vi "ManageGradientSearchRoutines.vi"(0 "System no.":i32=1 min=1 step=1, 5 "error in (no error)":errorcluster) -> (19 "error out":errorcluster)   [LabVIEW 2020]
doc: "This VI allows to add or edit Gradient Search Routines (FDG).\n\nRoutines can be managed on the controller directly or via text files."
uses:
  Message Cluster.ctl
  <vilib>/Utility/miscctls.llb/LVRowAndColumnTypeDef.ctl
panel:
  in  "Update from selected":bool
  in  "Name":string
  in  "Send to controller":bool
  in  "Board":i32 min=1 max=5 step=1
  in  "Minimum Level":dbl format="%.3f"
  in  "Speed offset":dbl format="%.4f"
  in  "Max. dir. changes":i32
  in  "Speed factor":dbl format="%.4f"
  in  "Max velocity":dbl format="%.4f"
  in  "Frequency":dbl format="%.3f"
  in  "Max amplitude":dbl format="%.4f"
  in  "Min amplitude":dbl format="%.4f"
  in  "Step axis":string
  in  "Scan axis":string
  in  "stop":bool
  in  "Available Routines":string[][](table)
  # "Routine definition"
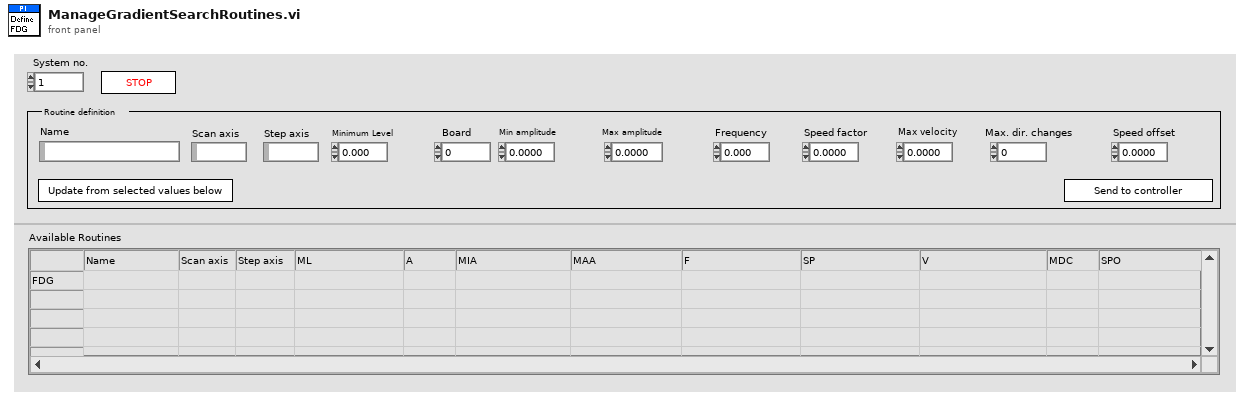
[diagram p1: front panel]
types:
  T1 = typedef "Message Cluster.ctl" = cluster{"Message":string, "Message Data":variant}
  T2 = cluster{"Set speed factor?":bool, "Speed factor":dbl}
  T3 = cluster{"Set max. velocity?":bool, "Max velocity":dbl}
  T4 = cluster{"Set max. dir. changes?":bool, "Max. dir. changes":i32}
  T5 = cluster{"Set speed offset?":bool, "Speed offset":dbl}
  T6 = cluster{"Min amplitude":dbl, "Set min. amplitude?":bool, "Max amplitude":dbl, "Set max. amplitude?":bool}
  T7 = typedef "LVRowAndColumnTypeDef.ctl" = cluster{"Row":i32, "Column":i32}
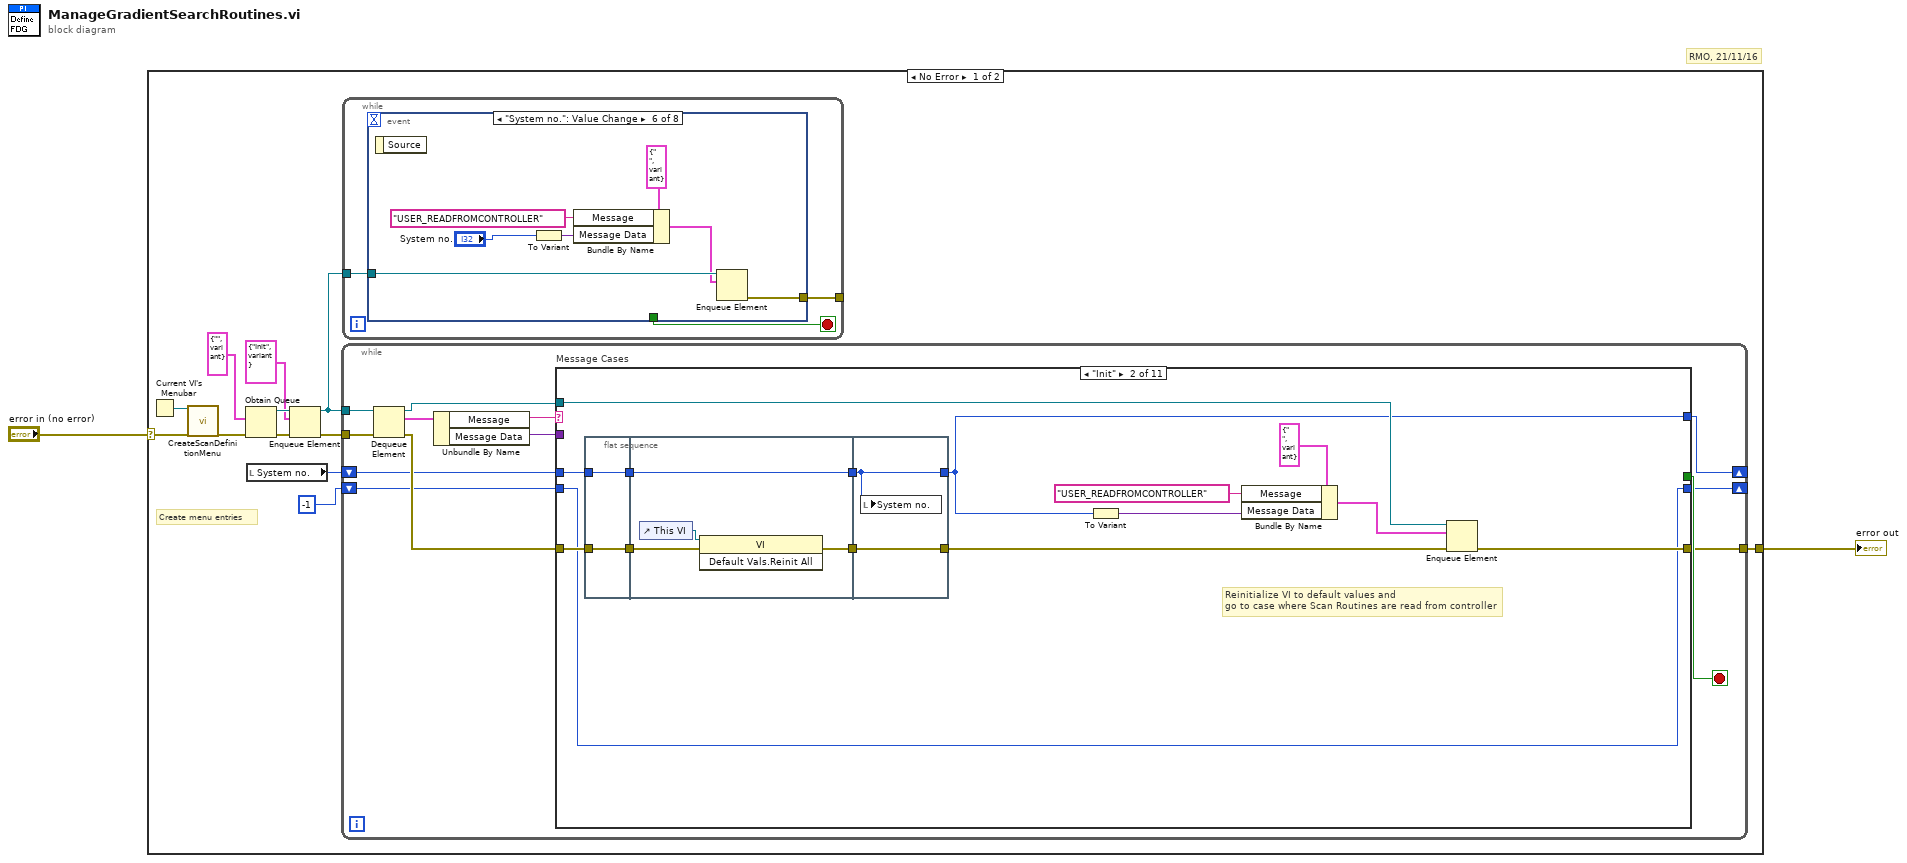
[diagram p0: block diagram]
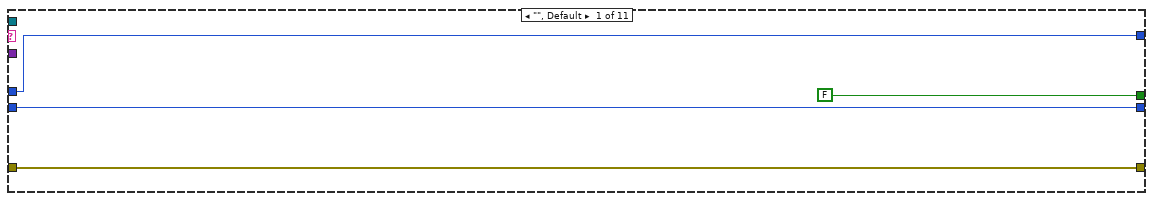
[diagram p2: hidden frame]
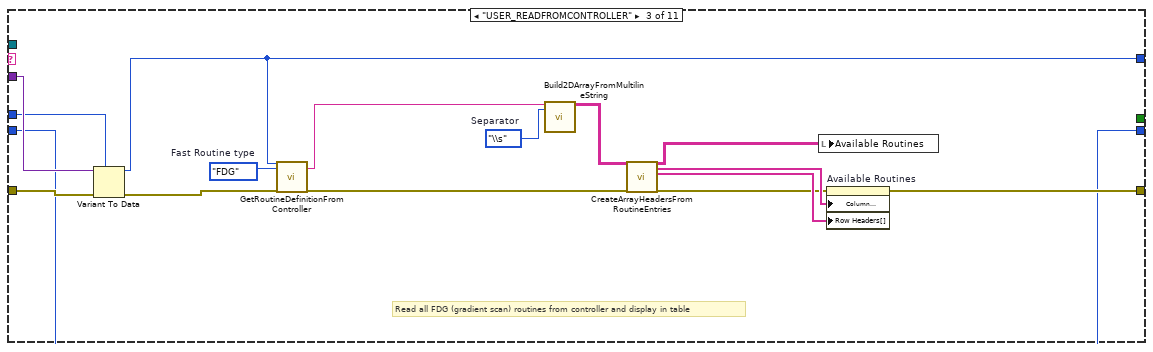
[diagram p3: hidden frame]
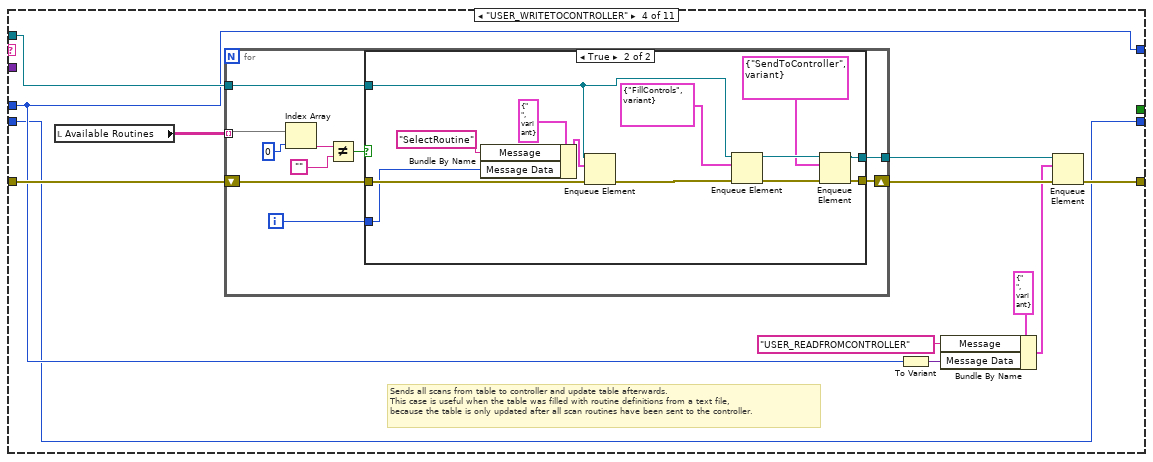
[diagram p4: hidden frame]
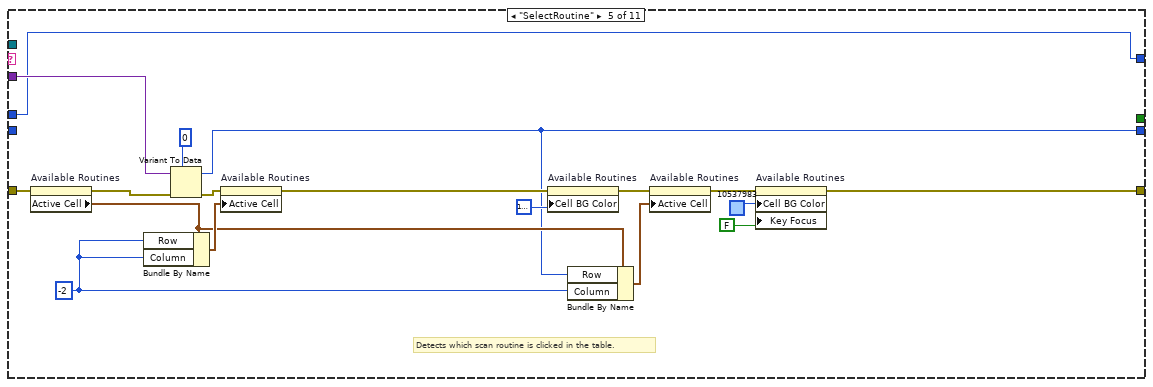
[diagram p6: hidden frame]
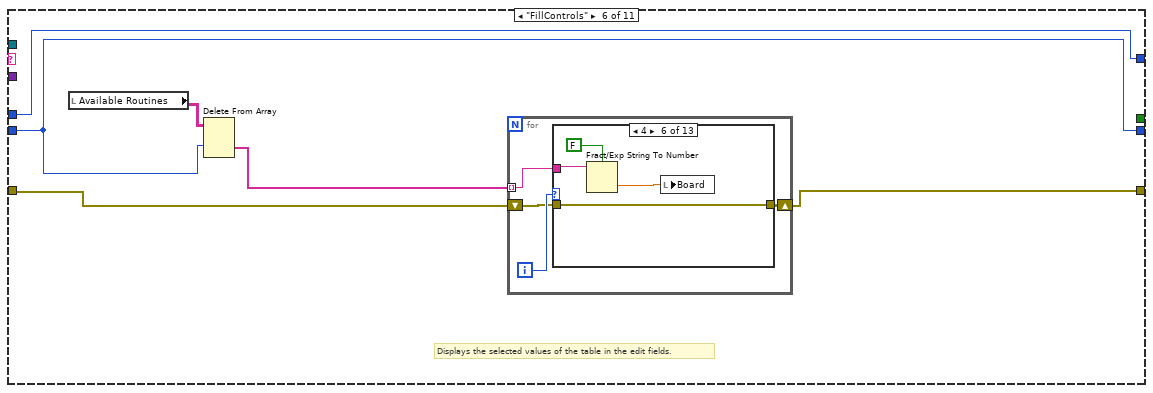
[diagram p7: hidden frame]
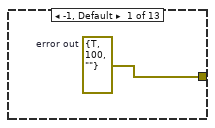
[diagram p8: hidden frame]
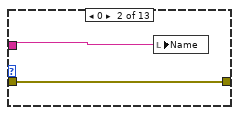
[diagram p9: hidden frame]
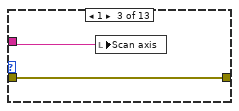
[diagram p10: hidden frame]
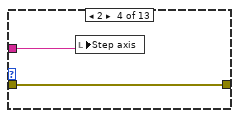
[diagram p11: hidden frame]
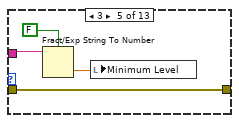
[diagram p12: hidden frame]
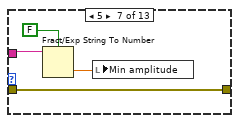
[diagram p13: hidden frame]
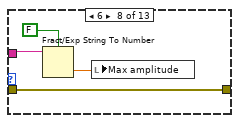
[diagram p14: hidden frame]
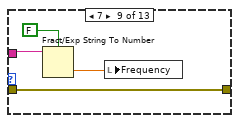
[diagram p15: hidden frame]
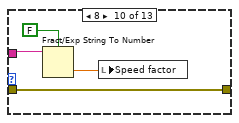
[diagram p16: hidden frame]
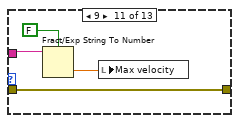
[diagram p17: hidden frame]
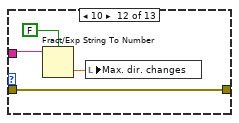
[diagram p18: hidden frame]
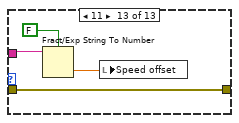
[diagram p19: hidden frame]
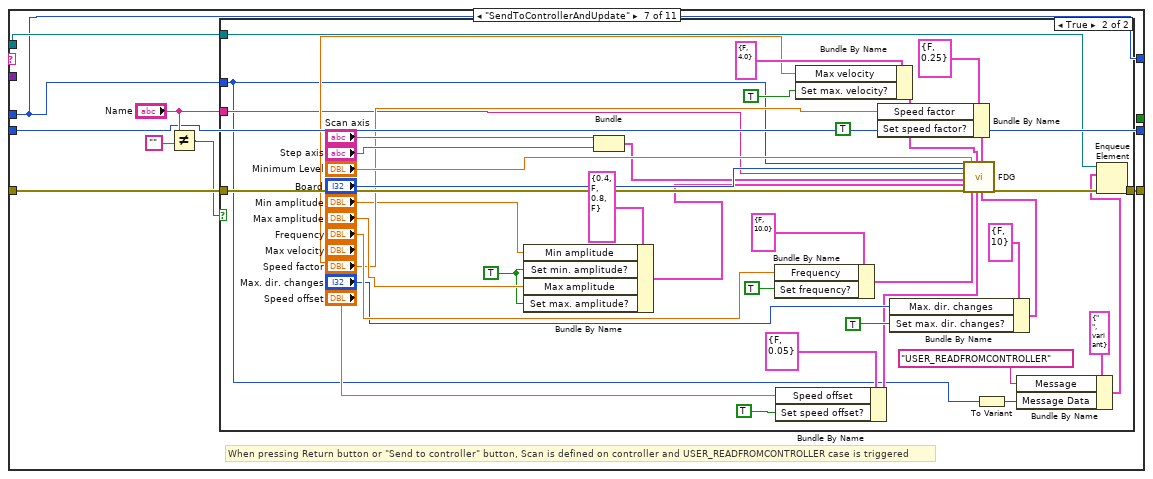
[diagram p20: hidden frame]
diagram:
  # "RMO, 21/11/16"
  n1 = case shown="No Error" "error in (no error)" {
    selector: "error in (no error)" -> [w5 w330]
    tunnel: [w6 w330] -> w2
    frame No Error {
      # "Create menu entries"
      n2 = Current VI's Menubar() -> (w7:refnum<k9>)
      n3 = call "CreateScanDefinitionMenu.vi"("menu reference"=w7, "error in (no error)"=w5) -> ("error out"=w8:errorcluster)  [unwired: 17 out]
      n4 = Obtain Queue(element data type=T1 {"Message"="", "Message Data"=variant} ("Message Cluster"), error in (no error)=w8) -> (queue out=w12:refnum<queue>, error out=w13:errorcluster)  [unwired: 2 in, 2 out]
      n5 = local read "System no."() -> (w4:i32)
      n6 = Enqueue Element(queue=w12, element=T1 {"Message"="Init", "Message Data"=variant}, error in (no error)=w13) -> (queue out=w9:refnum<queue>, error out=w10:errorcluster)  [unwired: 2 out]
      n7 = while {
        tunnel: w10 -> [w27]
        tunnel: w9 -> [w26]
        tunnel: [w21] -> w6
        shift-right: [w17] -> _
        shift-left: w4 -> [w20]
        shift-right: [w16] -> _
        shift-left: -1 ("Horizontal") -> [w15]
        stop <- w22 stop-if-true
        n8 = Dequeue Element(queue=w26, error in (no error)=w27) -> (queue out=w18:refnum<queue>, element=w25:T1, error out=w24:errorcluster)  [unwired: 2 out]
        n9 = Unbundle By Name(w25) -> ("Message"=w23:string, "Message Data"=w19:variant)
        n10 = case "Message Cases" shown="\"Init\"" w23 {
          tunnel: w24 -> [w31 w44 w61 w80 w123 w126 w186 w262 w268 w274 w286]
          tunnel: [w31 w45 w64 w78 w109 w129 w185 w242 w265 w276 w287] -> w21
          tunnel: [FALSE _ _ _ _ _ _ _ _ _ TRUE] -> w22
          tunnel: w20 -> [w29 w37 w58 w72 w110 w128 w180 w229 w264 w272 w283]
          tunnel: w19 -> [_ _ w59 _ w125 _ _ _ _ _ _]
          tunnel: w18 -> [_ w46 _ w81 _ _ w184 _ _ _ _]
          tunnel: [w29 w32 w57 w72 w110 w128 w180 w229 w264 w272 w283] -> w17
          tunnel: [w28 w38 w56 w71 w108 w127 w179 w228 w263 w271 w282] -> w16
          tunnel: w15 -> [w28 w38 w56 w71 _ w127 w179 w228 w263 w271 w282]
          frame "", Default {
          }
          frame "Init" {
            # "Reinitialize VI to default values and\ngo to case where Scan Routines are read from controller"
            n11 = flat-sequence {
              tunnel: w37 -> [w47]
              tunnel: w44 -> [w48]
              tunnel: [w48] -> w36
              tunnel: [w47] -> w35
              tunnel: w36 -> [w51]
              tunnel: w35 -> [w49]
              tunnel: [w50] -> w34
              tunnel: [w49] -> w33
              tunnel: [w54] -> w43
              tunnel: w34 -> [w54]
              tunnel: w33 -> [w53]
              tunnel: [w53] -> w32
              frame #0 {
              }
              frame #1 {
                n12 = control-ref of="This VI"() -> (w52:refnum<vi>)
                n13 = invoke class="VI" method="Default Vals.Reinit All"(reference=w52, error in=w51) -> (error out=w50:errorcluster)  [unwired: 1 in, 2 out]
              }
              frame #2 {
                n14 = local write "System no."(w53) -> ()
              }
            }
            n15 = To Variant(anything=w32) -> (Variant=w42:variant)
            n16 = Bundle By Name(cluster=T1 {"Message"="  ", "Message Data"=variant} ("Message Cluster"), "Message"="USER_READFROMCONTROLLER", "Message Data"=w42) -> (w39:T1)
            n17 = Enqueue Element(queue=w46, element=w39, error in (no error)=w43) -> (error out=w45:errorcluster)  [unwired: 3 out]
          }
          frame "USER_READFROMCONTROLLER" {
            w69 = enum16{"\\s", "\\t"}."\\s"  # Separator
            w70 = enum16{"FDG", "FDR"}."FDG"  # Fast Routine type
            # "Read all FDG (gradient scan) routines from controller and display in table"
            n18 = Variant To Data(error in=w61, type=w58, Variant=w59) -> (data=w57:i32, error out=w60:errorcluster)
            n19 = call "GetRoutineDefinitionFromController.vi"("System no."=w57, "Fast Routine type"=w70, "error in"=w60) -> ("Routine Definitons"=w55:string, "error out"=w63:errorcluster)  [unwired: 15 out]
            n20 = call "Build2DArrayFromMultilineString.vi"("String"=w55, "Separator"=w69) -> ("2D Array out"=w68:string[][])  [unwired: 17 out]
            n21 = call "CreateArrayHeadersFromRoutineEntries.vi"("Available Routines"=w68, "error in"=w63) -> ("Available Routines out"=w67:string[][], "Column Headers"=w66:string[], "Row Headers"=w65:string[], "error out"=w62:errorcluster)  [unwired: 14 out]
            n22 = local write "Available Routines"(w67) -> ()
            n23 = property on="Available Routines" class="Tbl (strict)"(error in=w62, "Column Headers[]"=w66, "Row Headers[]"=w65) -> (error out=w64:errorcluster)  [unwired: 1 in, 1 out]
          }
          frame "USER_WRITETOCONTROLLER" {
            # "Sends all scans from table to controller and update table afterwards.\nThis case is useful when the table was filled with routine definitions from a text file,\nbecause the table is only updated after all scan routines have been sent to the controller."
            n24 = local read "Available Routines"() -> (w82:string[][])
            n25 = for {
              tunnel: w82 -> [w88] mode=indexing
              tunnel: w81 -> [w91]
              shift-right: [w89] -> w79
              shift-left: w80 -> [w90]
              tunnel: [w83] -> w77
              i -> [w92]
              n26 = Index Array(array=w88, index=0) -> (element=w86:string)
              n27 = Not Equal?(x=w86, y="") -> (x != y?=w84:bool)
              n28 = case shown="True" w84 {
                tunnel: w92 -> [_ w96]
                tunnel: w91 -> [w93 w99]
                tunnel: w90 -> [w94 w101]
                tunnel: [w94 w103] -> w89
                tunnel: [w93 w102] -> w83
                frame False {
                }
                frame True {
                  n29 = Bundle By Name(cluster=T1 {"Message"="  ", "Message Data"=variant} ("Message Cluster"), "Message"="SelectRoutine", "Message Data"=w96) -> (w95:T1)
                  n30 = Enqueue Element(queue=w99, element=w95, error in (no error)=w101) -> (error out=w100:errorcluster)  [unwired: 3 out]
                  n31 = Enqueue Element(queue=w99, element=T1 {"Message"="FillControls", "Message Data"=variant} ("Message Cluster"), error in (no error)=w100) -> (queue out=w105:refnum<queue>, error out=w106:errorcluster)  [unwired: 2 out]
                  n32 = Enqueue Element(queue=w105, element=T1 {"Message"="SendToController", "Message Data"=variant}, error in (no error)=w106) -> (queue out=w102:refnum<queue>, error out=w103:errorcluster)  [unwired: 2 out]
                }
              }
            }
            n33 = To Variant(anything=w72) -> (Variant=w76:variant)
            n34 = Bundle By Name(cluster=T1 {"Message"="  ", "Message Data"=variant} ("Message Cluster"), "Message"="USER_READFROMCONTROLLER", "Message Data"=w76) -> (w74:T1)
            n35 = Enqueue Element(queue=w77, element=w74, error in (no error)=w79) -> (error out=w78:errorcluster)  [unwired: 3 out]
          }
          frame "SelectRoutine" {
            w115 = -2 ("Row")
            # "Detects which scan routine is clicked in the table."
            n36 = property on="Available Routines" class="Tbl (strict)"(error in=w123) -> (error out=w111:errorcluster, "Active Cell"=w116:T7)  [unwired: 1 in, 1 out]
            n37 = Bundle By Name(cluster=w116, "Row"=w115, "Column"=w115) -> (w120:T7)
            n38 = Variant To Data(error in=w111, type=0 ("Horizontal"), Variant=w125) -> (data=w108:i32, error out=w122:errorcluster)
            n39 = property on="Available Routines" class="Tbl (strict)"(error in=w122, "Active Cell"=w120) -> (error out=w121:errorcluster)  [unwired: 1 in, 1 out]
            n40 = property on="Available Routines" class="Tbl (strict)"(error in=w121, "Cell BG Color"=u32 16777225 ("Color Box")) -> (error out=w119:errorcluster)  [unwired: 1 in, 1 out]
            n41 = Bundle By Name(cluster=w116, "Row"=w108, "Column"=w115) -> (w114:T7)
            n42 = property on="Available Routines" class="Tbl (strict)"(error in=w119, "Active Cell"=w114) -> (error out=w118:errorcluster)  [unwired: 1 in, 1 out]
            n43 = property on="Available Routines" class="Tbl (strict)"(error in=w118, "Cell BG Color"=u32 10537983 ("Color Box"), "Key Focus"=FALSE) -> (error out=w109:errorcluster)  [unwired: 1 in, 1 out]
          }
          frame "FillControls" {
            # "Displays the selected values of the table in the edit fields."
            n44 = local read "Available Routines"() -> (w131:string[][])
            n45 = Delete From Array(array=w131, index (row)=w127) -> (deleted portion=w130:string[])  [unwired: 2 in, 1 out]
            n46 = for {
              tunnel: w130 -> [w135] mode=indexing
              shift-right: [w132] -> w129
              shift-left: w126 -> [w133]
              i -> [w134]
              n47 = case shown="4" w134 {
                tunnel: w135 -> [_ w137 w140 w142 w145 w149 w153 w157 w161 w165 w169 w173 w177]
                tunnel: w133 -> [_ w138 w139 w141 w146 w150 w154 w158 w162 w166 w170 w174 w178]
                tunnel: [w136 w138 w139 w141 w146 w150 w154 w158 w162 w166 w170 w174 w178] -> w132
                frame -1, Default {
                  w136 = errorcluster {"status"=TRUE, "code"=100, "source"=""}  # error out
                }
                frame 0 {
                  n48 = local write "Name"(w137) -> ()
                }
                frame 1 {
                  n49 = local write "Scan axis"(w140) -> ()
                }
                frame 2 {
                  n50 = local write "Step axis"(w142) -> ()
                }
                frame 3 {
                  n51 = Fract/Exp String To Number(use system decimal point (T)=FALSE, string=w145) -> (number=w144:dbl)  [unwired: 3 out]
                  n52 = local write "Minimum Level"(w144) -> ()
                }
                frame 4 {
                  n53 = Fract/Exp String To Number(use system decimal point (T)=FALSE, string=w149) -> (number=w148:dbl)  [unwired: 3 out]
                  n54 = local write "Board"(w148) -> ()
                }
                frame 5 {
                  n55 = Fract/Exp String To Number(use system decimal point (T)=FALSE, string=w153) -> (number=w152:dbl)  [unwired: 3 out]
                  n56 = local write "Min amplitude"(w152) -> ()
                }
                frame 6 {
                  n57 = Fract/Exp String To Number(use system decimal point (T)=FALSE, string=w157) -> (number=w156:dbl)  [unwired: 3 out]
                  n58 = local write "Max amplitude"(w156) -> ()
                }
                frame 7 {
                  n59 = Fract/Exp String To Number(use system decimal point (T)=FALSE, string=w161) -> (number=w160:dbl)  [unwired: 3 out]
                  n60 = local write "Frequency"(w160) -> ()
                }
                frame 8 {
                  n61 = Fract/Exp String To Number(use system decimal point (T)=FALSE, string=w165) -> (number=w164:dbl)  [unwired: 3 out]
                  n62 = local write "Speed factor"(w164) -> ()
                }
                frame 9 {
                  n63 = Fract/Exp String To Number(use system decimal point (T)=FALSE, string=w169) -> (number=w168:dbl)  [unwired: 3 out]
                  n64 = local write "Max velocity"(w168) -> ()
                }
                frame 10 {
                  n65 = Fract/Exp String To Number(use system decimal point (T)=FALSE, string=w173) -> (number=w172:dbl)  [unwired: 3 out]
                  n66 = local write "Max. dir. changes"(w172) -> ()
                }
                frame 11 {
                  n67 = Fract/Exp String To Number(use system decimal point (T)=FALSE, string=w177) -> (number=w176:dbl)  [unwired: 3 out]
                  n68 = local write "Speed offset"(w176) -> ()
                }
              }
            }
          }
          frame "SendToControllerAndUpdate" {
            # "When pressing Return button or \"Send to controller\" button, Scan is defined on controller and USER_READFROMCONTROLLER case is triggered"
            n69 = Not Equal?(x="Name", y="") -> (x != y?=w182:bool)
            n70 = case shown="True" w182 {
              tunnel: w186 -> [w187 w227]
              tunnel: w180 -> [_ w188]
              tunnel: [w187 w196] -> w185
              tunnel: w184 -> [_ w195]
              tunnel: "Name" -> [_ w193]
              frame False {
              }
              frame True {
                w218 = TRUE
                n71 = Bundle By Name(cluster=T6 {"Min amplitude"=0.4, "Set min. amplitude?"=FALSE, "Max amplitude"=0.8, "Set max. amplitude?"=FALSE} ("Amplitude settings"), "Min amplitude"="Min amplitude", "Set min. amplitude?"=w218, "Max amplitude"="Max amplitude", "Set max. amplitude?"=w218) -> (w220:T6)
                n72 = Bundle("Scan axis"="Scan axis", "Step axis"="Step axis") -> (w222:cluster{"Scan axis":string, "Step axis":string})  [unwired: 1 out]
                n73 = Bundle By Name(cluster=cluster{"Set frequency?":bool, "Frequency":dbl} {"Set frequency?"=FALSE, "Frequency"=10.0} ("Frequency settings"), "Frequency"="Frequency", "Set frequency?"=TRUE) -> (w216:cluster{"Set frequency?":bool, "Frequency":dbl})
                n74 = Bundle By Name(cluster=T5 {"Set speed offset?"=FALSE, "Speed offset"=0.05} ("Speed offset settings"), "Speed offset"="Speed offset", "Set speed offset?"=TRUE) -> (w207:T5)
                n75 = Bundle By Name(cluster=T3 {"Set max. velocity?"=FALSE, "Max velocity"=4.0} ("Velocity settings"), "Max velocity"="Max velocity", "Set max. velocity?"=TRUE) -> (w203:T3)
                n76 = Bundle By Name(cluster=T2 {"Set speed factor?"=FALSE, "Speed factor"=0.25} ("Speed factor settings"), "Speed factor"="Speed factor", "Set speed factor?"=TRUE) -> (w204:T2)
                n77 = Bundle By Name(cluster=T4 {"Set max. dir. changes?"=FALSE, "Max. dir. changes"=10} ("Max. direction changes settings"), "Max. dir. changes"="Max. dir. changes", "Set max. dir. changes?"=TRUE) -> (w213:T4)
                n78 = call "FDG.vi"("System no."=w188, "Board"="Board", "Routinename"=w193, "Axis settings"=w222, "Amplitude settings"=w220, "error in"=w227, "Minimum Level"="Minimum Level", "Frequency settings"=w216, "Velocity settings"=w203, "Speed offset settings"=w207, "Speed factor settings"=w204, "Max. direction changes settings"=w213) -> ("error out"=w197:errorcluster)  [unwired: 7 out]
                n79 = To Variant(anything=w188) -> (Variant=w190:variant)
                n80 = Bundle By Name(cluster=T1 {"Message"="  ", "Message Data"=variant} ("Message Cluster"), "Message"="USER_READFROMCONTROLLER", "Message Data"=w190) -> (w189:T1)
                n81 = Enqueue Element(queue=w195, element=w189, error in (no error)=w197) -> (error out=w196:errorcluster)  [unwired: 3 out]
              }
            }
          }
          frame "SendToController" {
            w258 = TRUE
            # "Defines gradient scan routine on controller."
            n82 = local read "Max. dir. changes"() -> (w232:i32)
            n83 = local read "Minimum Level"() -> (w239:dbl)
            n84 = local read "Max amplitude"() -> (w236:dbl)
            n85 = local read "Min amplitude"() -> (w237:dbl)
            n86 = local read "Max velocity"() -> (w234:dbl)
            n87 = local read "Speed factor"() -> (w233:dbl)
            n88 = local read "Speed offset"() -> (w231:dbl)
            n89 = local read "Frequency"() -> (w235:dbl)
            n90 = local read "Scan axis"() -> (w241:string)
            n91 = local read "Step axis"() -> (w240:string)
            n92 = local read "Name"() -> (w230:string)
            n93 = local read "Board"() -> (w238:i32)
            n94 = Bundle By Name(cluster=T6 {"Min amplitude"=0.4, "Set min. amplitude?"=FALSE, "Max amplitude"=0.8, "Set max. amplitude?"=FALSE} ("Amplitude settings"), "Min amplitude"=w237, "Set min. amplitude?"=w258, "Max amplitude"=w236, "Set max. amplitude?"=w258) -> (w259:T6)
            n95 = Bundle("Scan axis"=w241, "Step axis"=w240) -> (w261:cluster{"Scan axis":string, "Step axis":string})  [unwired: 1 out]
            n96 = Bundle By Name(cluster=cluster{"Set frequency?":bool, "Frequency":dbl} {"Set frequency?"=FALSE, "Frequency"=10.0} ("Frequency settings"), "Frequency"=w235, "Set frequency?"=TRUE) -> (w256:cluster{"Set frequency?":bool, "Frequency":dbl})
            n97 = Bundle By Name(cluster=T5 {"Set speed offset?"=FALSE, "Speed offset"=0.05} ("Speed offset settings"), "Speed offset"=w231, "Set speed offset?"=TRUE) -> (w250:T5)
            n98 = Bundle By Name(cluster=T3 {"Set max. velocity?"=FALSE, "Max velocity"=4.0} ("Velocity settings"), "Max velocity"=w234, "Set max. velocity?"=TRUE) -> (w246:T3)
            n99 = Bundle By Name(cluster=T2 {"Set speed factor?"=FALSE, "Speed factor"=0.25} ("Speed factor settings"), "Speed factor"=w233, "Set speed factor?"=TRUE) -> (w247:T2)
            n100 = Bundle By Name(cluster=T4 {"Set max. dir. changes?"=FALSE, "Max. dir. changes"=10} ("Max. direction changes settings"), "Max. dir. changes"=w232, "Set max. dir. changes?"=TRUE) -> (w254:T4)
            n101 = call "FDG.vi"("System no."=w229, "Board"=w238, "Routinename"=w230, "Axis settings"=w261, "Amplitude settings"=w259, "error in"=w262, "Minimum Level"=w239, "Frequency settings"=w256, "Velocity settings"=w246, "Speed offset settings"=w250, "Speed factor settings"=w247, "Max. direction changes settings"=w254) -> ("error out"=w242:errorcluster)  [unwired: 7 out]
          }
          frame "USER_SAVETOFILE" {
            w269 = enum16{"FDG", "FDR"}."FDG"  # Fast Routine type
            # "Saves all FDG routines to text file."
            n102 = call "GetRoutineDefinitionFromController.vi"("System no."=w264, "Fast Routine type"=w269, "error in"=w268) -> ("Routine Definitons"=w266:string, "error out"=w267:errorcluster)  [unwired: 15 out]
            n103 = Write to Text File(text=w266, error in=w267) -> (error out=w265:errorcluster)  [unwired: 4 out]
          }
          frame "USER_LOADFROMFILE" {
            w281 = enum16{"\\s", "\\t"}."\\s"  # Separator
            # "Load all gradient scan routines from text file and display in table"
            n104 = Read from Text File(error in=w274) -> (text=w270:string, error out=w273:errorcluster)  [unwired: 5 out]
            n105 = call "Build2DArrayFromMultilineString.vi"("String"=w270, "Separator"=w281) -> ("2D Array out"=w280:string[][])  [unwired: 17 out]
            n106 = call "CreateArrayHeadersFromRoutineEntries.vi"("Available Routines"=w280, "error in"=w273) -> ("Available Routines out"=w279:string[][], "Column Headers"=w278:string[], "Row Headers"=w277:string[], "error out"=w275:errorcluster)  [unwired: 14 out]
            n107 = local write "Available Routines"(w279) -> ()
            n108 = property on="Available Routines" class="Tbl (strict)"(error in=w275, "Column Headers[]"=w278, "Row Headers[]"=w277) -> (error out=w276:errorcluster)  [unwired: 1 in, 1 out]
          }
          frame "Exit" {
            w284 = T7 {"Row"=0, "Column"=0} ("Selection Start")
            n109 = property on="Available Routines" class="Tbl (strict)"(error in=w286, "Selection Start"=w284, "Selection Size"=w284) -> (error out=w285:errorcluster)  [unwired: 1 in, 1 out]
            n110 = property on="Available Routines" class="Tbl (strict)"(error in=w285, "Cell BG Color"=u32 16777225 ("Color Box")) -> (error out=w287:errorcluster)  [unwired: 1 in, 1 out]
          }
        }
      }
      n111 = while {
        tunnel: w9 -> [w292]
        tunnel: [w291] -> _
        stop <- w290 stop-if-true
        n112 = event shown="[5] \"System no.\": Value Change" {
          selector: _ -> [_ _ _ _ _ _ _ _]
          dyn-events: _ -> [_ _ _ _ _ _ _ _]
          timeout: _ -> [_ _ _ _ _ _ _ _]
          tunnel: w292 -> [_ w295 w300 w304 w316 w322 w326 w327]
          tunnel: [_ w293 w298 w303 w315 w323 w325 w328] -> w291
          tunnel: [_ "stop" TRUE _ _ _ _ _] -> w290
          event Timeout {
            n113 = event-data() -> ()  [unwired: 3 out]
          }
          event "stop": Value Change {
            n114 = event-data() -> ()  [unwired: 5 out]
            n115 = Enqueue Element(queue=w295, element=T1 {"Message"="Exit", "Message Data"=variant}) -> (error out=w293:errorcluster)  [unwired: 1 in, 3 out]
          }
          event Panel Close? {
            n116 = event-data() -> ()  [unwired: 5 out]
            n117 = Enqueue Element(queue=w300, element=T1 {"Message"="Exit", "Message Data"=variant}) -> (error out=w298:errorcluster)  [unwired: 1 in, 3 out]
            n118 = event-data() -> ()  [unwired: 1 in, 2 out]
          }
          event Menu Selection (User) {
            n119 = event-data() -> ("ItemTag"=w306:string)  [unwired: 1 out]
            n120 = local read "System no."() -> (w301:i32)
            n121 = To Variant(anything=w301) -> (Variant=w302:variant)
            n122 = Bundle By Name(cluster=T1 {"Message"="", "Message Data"=variant} ("Message Cluster"), "Message"=w306, "Message Data"=w302) -> (w305:T1)
            n123 = Enqueue Element(queue=w304, element=w305) -> (error out=w303:errorcluster)  [unwired: 1 in, 3 out]
          }
          event "Available Routines": Mouse Down {
            n124 = event-data() -> ("CtlRef"=w310:refnum<vi>)  [unwired: 1 out]
            n125 = property class="Tbl (strict)"(reference=w310) -> ("Selection Start"=w309:T7)  [unwired: 1 in, 2 out]
            n126 = Unbundle By Name(w309) -> ("Row"=w308:i32)
            n127 = To Variant(anything=w308) -> (Variant=w312:variant)
            n128 = Bundle By Name(cluster=T1 {"Message"="  ", "Message Data"=variant} ("Message Cluster"), "Message"="SelectRoutine", "Message Data"=w312) -> (w311:T1)
            n129 = Enqueue Element(queue=w316, element=w311) -> (error out=w315:errorcluster)  [unwired: 1 in, 3 out]
          }
          event "System no.": Value Change {
            n130 = event-data() -> ()  [unwired: 2 out]
            n131 = To Variant(anything="System no.") -> (Variant=w319:variant)
            n132 = Bundle By Name(cluster=T1 {"Message"="  ", "Message Data"=variant} ("Message Cluster"), "Message"="USER_READFROMCONTROLLER", "Message Data"=w319) -> (w317:T1)
            n133 = Enqueue Element(queue=w322, element=w317) -> (error out=w323:errorcluster)  [unwired: 1 in, 3 out]
          }
          event "Send to controller": Value Change; "Send to controller": Key Down {
            n134 = event-data() -> ()  [unwired: 5 out]
            n135 = Enqueue Element(queue=w326, element=T1 {"Message"="SendToControllerAndUpdate", "Message Data"=variant}) -> (error out=w325:errorcluster)  [unwired: 1 in, 3 out]
          }
          event "Update from selected": Value Change {
            n136 = event-data() -> ()  [unwired: 2 out]
            n137 = Enqueue Element(queue=w327, element=T1 {"Message"="FillControls", "Message Data"=variant} ("Message Cluster")) -> (error out=w328:errorcluster)  [unwired: 1 in, 3 out]
          }
        }
      }
    }
    frame Error {
    }
  }
  "error out" <- w2
